vi "test.PushPopNumber.vi"() -> ()   [LabVIEW 2014]
uses:
  Private/Class/class.GLue.lvclass
panel:
  out "*(type *) &x 2":u64
  out "*(type *) &x":u64
  out "Number":dbl format="%#.10f"
  out "error out":errorcluster
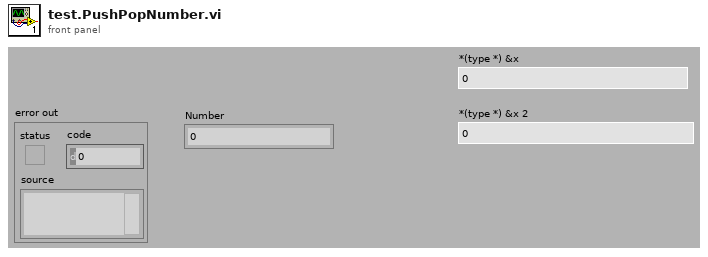
[diagram p1: front panel]
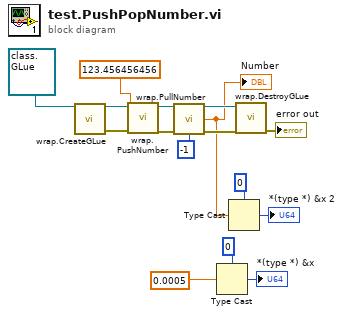
[diagram p0: block diagram]
diagram:
  n1 = call "wrap.CreateGLue.vi"("class.GLue in"=refnum<class "class.GLue.lvclass"> refnum) -> ("class.GLue out"=w15:refnum<class "class.GLue.lvclass">, "error out"=w16:errorcluster)  [unwired: 13 in]
  n2 = call "wrap.PushNumber.vi"("class.GLue in"=w15, "Numeric"=123.456456456, "error in (no error)"=w16) -> ("class.GLue out"=w12:refnum<class "class.GLue.lvclass">, "error out"=w13:errorcluster)  [unwired: 11 in]
  n3 = call "wrap.PullNumber.vi"("class.GLue in"=w12, "error in (no error)"=w13, "Index"=-1) -> ("class.GLue out"=w8:refnum<class "class.GLue.lvclass">, "Number"=w2:dbl, "error out"=w10:errorcluster)  [unwired: 10 in]
  "Number" <- w2
  n4 = Type Cast(type=u64 0, x=0.0005) -> (*(type *) &x=→"*(type *) &x":u64)
  n5 = Type Cast(type=u64 0, x=w2) -> (*(type *) &x=→"*(type *) &x 2":u64)
  n6 = call "wrap.DestroyGLue.vi"("class.GLue in"=w8, "error in (no error)"=w10) -> ("error out"=→"error out":errorcluster)  [unwired: 12 in, 1 out]
